vi "TazeASharg.vi"() -> ()   [LabVIEW 2022 SP3]
uses:
  ShargStates.ctl
  ShargTypeDef.ctl
  <vilib>/numeric/Random Number (Range) U64.vi
  <vilib>/numeric/sub_Random U32.vi
  <vilib>/MakerHub/LINX/Public/Utilities/Open Serial.vi
  <vilib>/MakerHub/LINX/Public/Sensors/Motion/Servo/Servo Open One Channel.vi
  <vilib>/MakerHub/LINX/Public/Sensors/Motion/Servo/Servo Close One Channel.vi
  <vilib>/MakerHub/LINX/LMH-LINX.lvlib
  <vilib>/MakerHub/LINX/Public/Sensors/Motion/Servo/Servo.lvlib
panel:
  out "High Scores":string[][](array[string])
  in  "Name":string
  out "Energy":dbl(slide) scale=0.0..100.0
  out "Overheat":bool
  out "Combo":u32
  out "Time":u32
  out "Hit?":bool
  out "Error Out":errorcluster
  out "Cluster Out":T1
  out "Live Score":u32
  out "State":T2=enum."Leaderboard"
  in  "Start Game":bool
  in  "Stop Button":bool
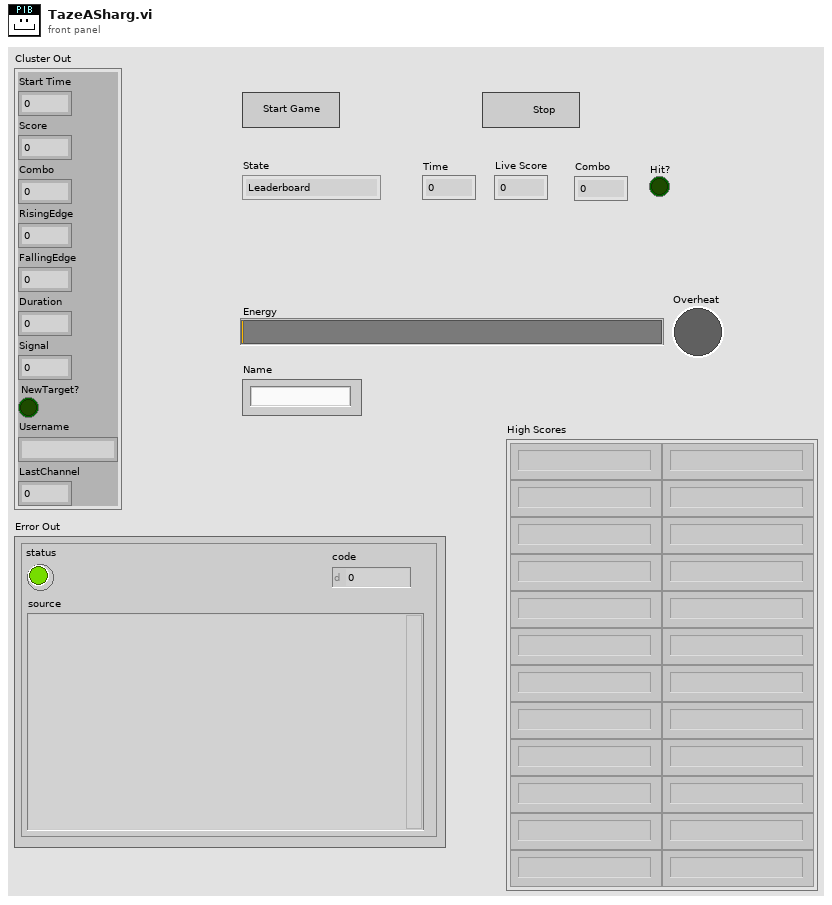
[diagram p1: front panel]
types:
  T1 = typedef "ShargTypeDef.ctl" = cluster{"Start Time":u32, "Score":u32, "Combo":u32, "RisingEdge":u32, "FallingEdge":u32, "Duration":u32, "Signal":i16, "NewTarget?":bool, "Username":string, "LastChannel":i32}
  T2 = typedef "ShargStates.ctl" = enum16{"Initialization", "Leaderboard", "Start Game", "Gameplay", "Update Final Score"}
  T3 = cluster{"Target Up":bool, "Target Start Time":u32, "Target Up Time":u64, "Current Target":u64}
  T4 = cluster{"Laser Pin":u8, "Trigger Pin":u8, "Servo Pin":u8, "Photoresistor Pins":u8[], "RGB LED Pins":u8[]}
  T5 = typedef "LMH-LINX.lvlib/LINX Ref.ctl" = cluster{"IO":T6, "Interface":T7, "LINX Device Config":T8}
  T6 = typedef "LMH-LINX.lvlib/Platform.ctl" = enum16{"Remote", "Local"}
  T7 = typedef "LMH-LINX.lvlib/Interface.ctl" = enum16{"Serial", "TCP"}
  T8 = typedef "LMH-LINX.lvlib/Device.lvlib/LINX Device Config.ctl" = cluster{"Interface":T7, "COM Port":refnum<visa-resource-name>, "TCP Configuration":T9, "Device Family":u8, "Device ID":u8, "Device Name":string, "TCP Ref":refnum<k5>, "Channels":T10}
  T9 = typedef "LMH-LINX.lvlib/Device.lvlib/TCP Config.ctl" = cluster{"IP Address":string, "Port":u16}
  T10 = typedef "LMH-LINX.lvlib/Channels.ctl" = cluster{"DI":u8[], "DO":u8[], "AI":u8[], "AO":u8[], "PWM":u8[], "QE":u8[], "UART":u8[], "I2C 2":u8[], "SPI":u8[], "CAN":u8[], "Servo":u8[], "AI Ref (V)":dbl, "AI Resolution (Bits)":u8, "AO Ref (V)":dbl, "AO Resolution (Bits)":u8}
  T11 = cluster{"Target Up":bool, "millisecond timer value":u32, "number":u64, "Current Target":u64}
  T12 = cluster{"Live Score":u32, "Time":u32, "Combo":u32}
  T13 = enum16{"open", "open or create", "create or replace", "create", "open (read-only)"}
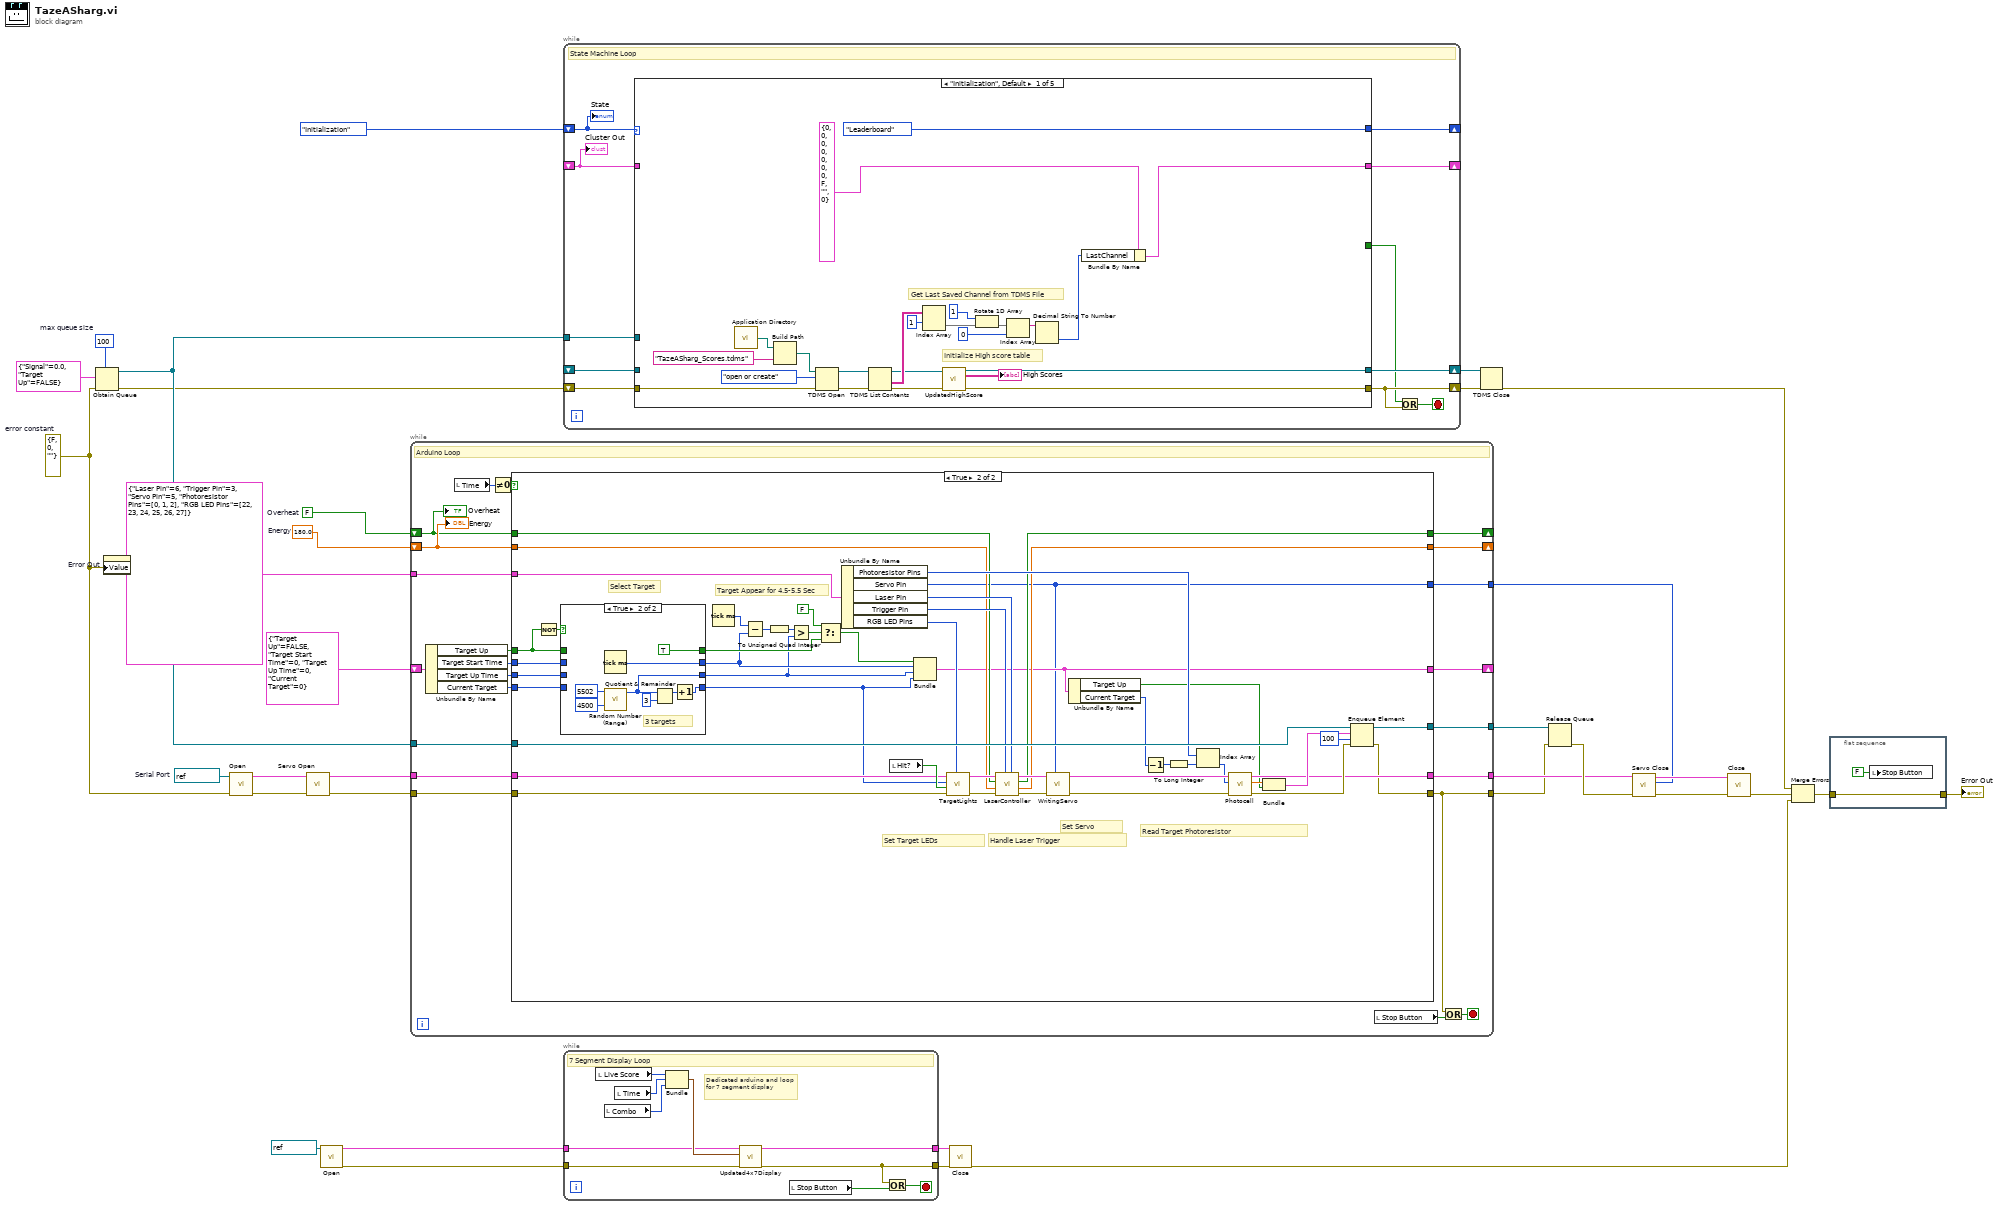
[diagram p0: block diagram]
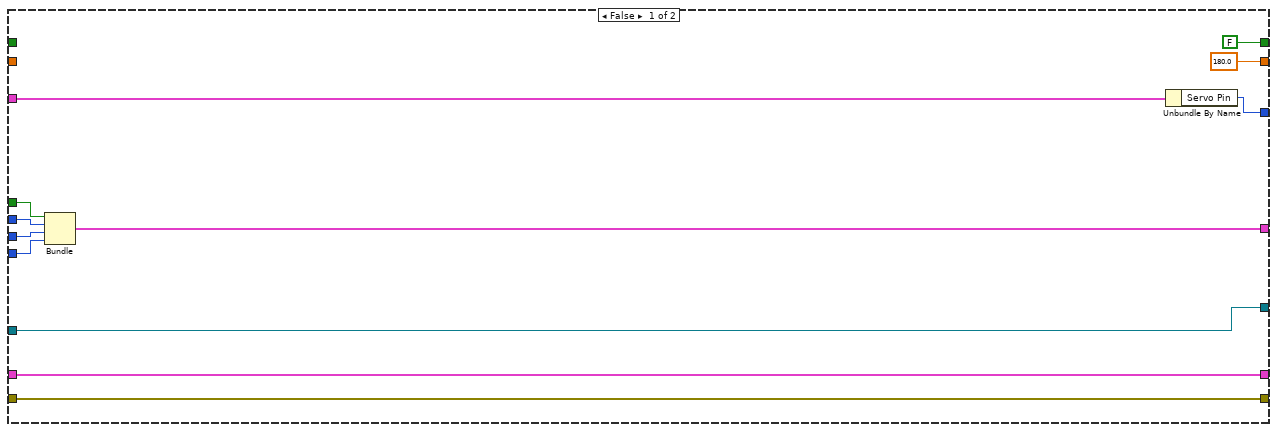
[diagram p2: hidden frame]
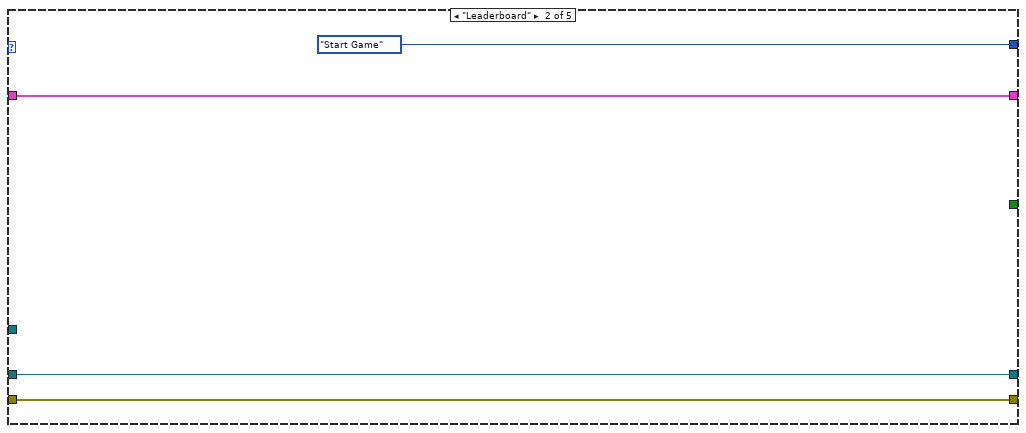
[diagram p4: hidden frame]
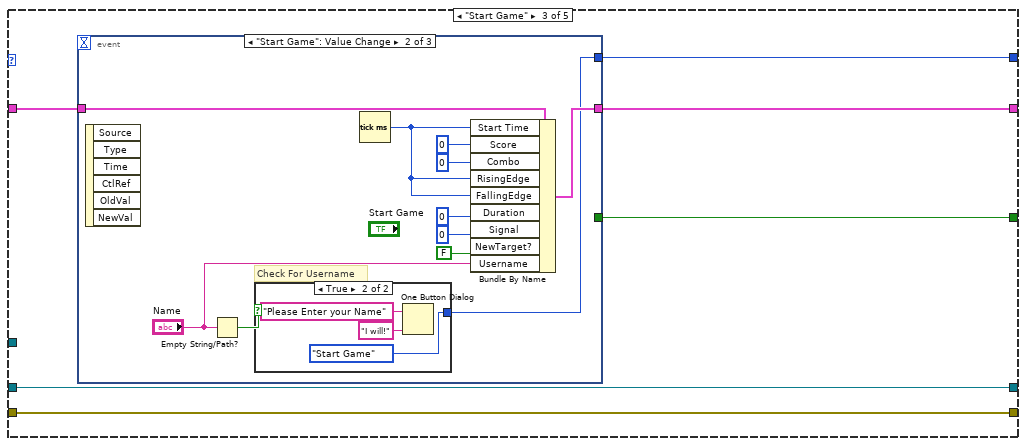
[diagram p5: hidden frame]
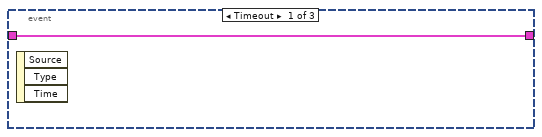
[diagram p6: hidden frame]
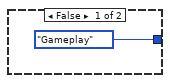
[diagram p7: hidden frame]
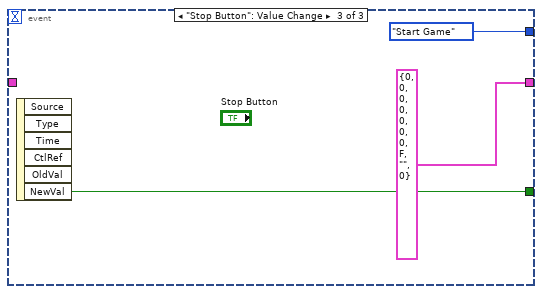
[diagram p8: hidden frame]
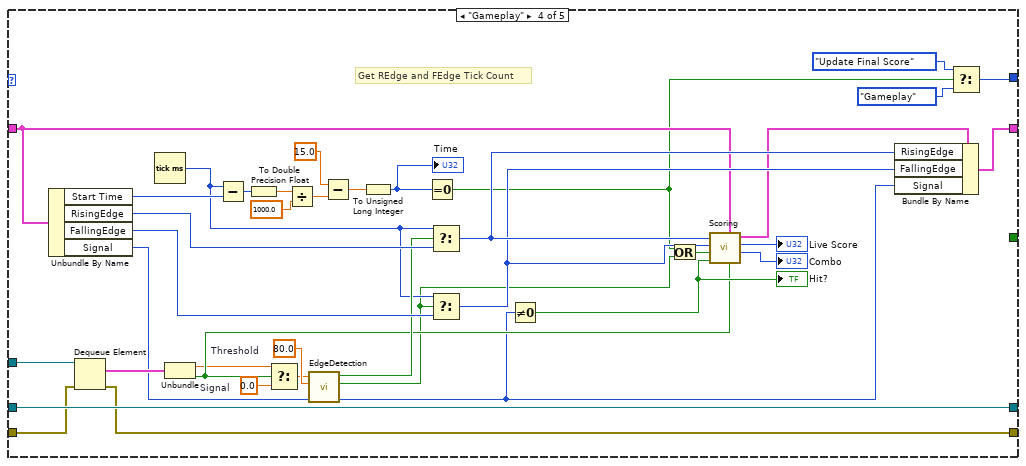
[diagram p9: hidden frame]
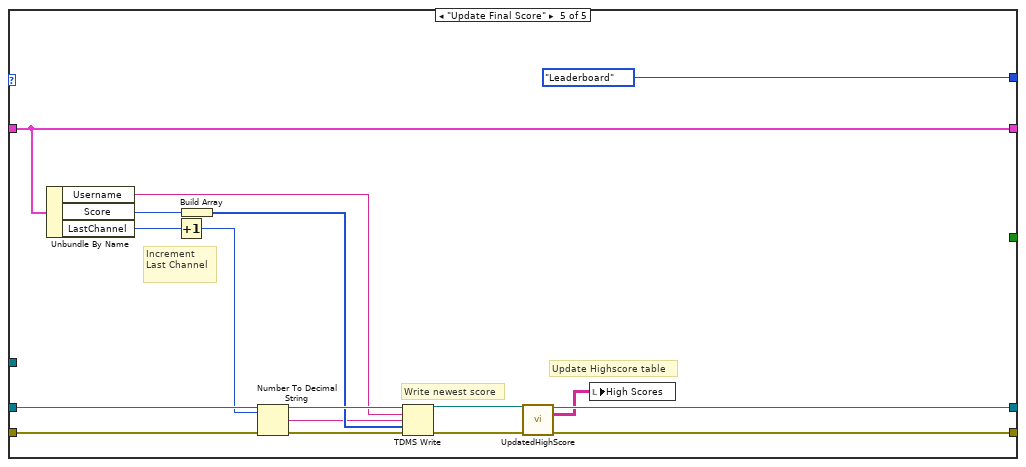
[diagram p10: hidden frame]
diagram:
  w6 = 180.0  # Energy
  w7 = FALSE  # Overheat
  w30 = refnum<visa-resource-name> "COM8"  # Serial Port
  w31 = 100  # max queue size
  w9 = errorcluster {"status"=FALSE, "code"=0, "source"=""}  # error constant
  n1 = Obtain Queue(max queue size (-1, unlimited)=w31, element data type=cluster{"Signal":dbl, "Target Up":bool} {"Signal"=0.0, "Target Up"=FALSE}, error in (no error)=w9) -> (queue out=w33:refnum<queue>, error out=w10:errorcluster)  [unwired: 2 in, 1 out]
  n2 = property on="Error Out" class="Clust (strict)"("Value"=w9) -> ()  [unwired: 2 in, 2 out]
  n3 = call-poly <vilib>:"Open.vi"("Error In"=w9, "Serial Port"=w30) -> ("Error Out"=w27:errorcluster, "LINX Resource"=w29:T5)  [unwired: 7 in, 1 out]
  n4 = call-poly <vilib>:"Servo Open.vi"("Error In"=w27, "LINX Resource"=w29) -> ("Error Out"=w26:errorcluster, "LINX Resource"=w28:T5)  [unwired: 8 in]
  n5 = call-poly <vilib>:"Open.vi"("Serial Port"=refnum<visa-resource-name> "COM5") -> ("Error Out"=w19:errorcluster, "LINX Resource"=w20:T5)  [unwired: 8 in, 1 out]
  n6 = while {
    tunnel: w26 -> [w51]
    tunnel: w28 -> [w52]
    shift-right: [w48] -> _
    shift-left: w7 -> [w45]
    shift-right: [w47] -> _
    shift-left: w6 -> [w46]
    tunnel: w33 -> [w50]
    tunnel: T4 {"Laser Pin"=6, "Trigger Pin"=3, "Servo Pin"=5, "Photoresistor Pins"=[0, 1, 2], "RGB LED Pins"=[22, 23, 24, 25, 26, 27]} -> [w49]
    tunnel: [w44] -> w5
    tunnel: [w35] -> w1
    tunnel: [w43] -> w4
    shift-right: [w37] -> _
    shift-left: T3 {"Target Up"=FALSE, "Target Start Time"=0, "Target Up Time"=0, "Current Target"=0} -> [w42]
    tunnel: [w36] -> w2
    stop <- w54 stop-if-true
    # "Arduino Loop"
    n7 = Unbundle By Name(w42) -> ("Target Up"=w41:bool, "Target Start Time"=w40:u32, "Target Up Time"=w39:u64, "Current Target"=w38:u64)
    n8 = local read "Time"() -> (w56:u32)
    n9 = Not Equal To 0?(x=w56) -> (x != 0?=w55:bool)
    n10 = case shown="True" w55 {
      tunnel: w40 -> [w62 w111]
      tunnel: w41 -> [w63 w110]
      tunnel: w38 -> [w60 w109]
      tunnel: w39 -> [w61 w108]
      tunnel: w52 -> [w65 w92]
      tunnel: w51 -> [w66 w91]
      tunnel: [w65 w90] -> w44
      tunnel: [w66 w89] -> w35
      tunnel: w50 -> [w64 w88]
      tunnel: w49 -> [w58 w86]
      tunnel: w46 -> [_ w81]
      tunnel: w45 -> [_ w80]
      tunnel: [FALSE ("Overheat Out") w79] -> w48
      tunnel: [180.0 ("Energy Out") w78] -> w47
      tunnel: [w64 w77] -> w43
      tunnel: [w59 w72] -> w37
      tunnel: [w57 w70] -> w36
      frame False {
        n11 = Bundle("Target Up"=w63, "Target Start Time"=w62, "Target Up Time"=w61, "Current Target"=w60) -> (w59:T3)  [unwired: 1 in]
        n12 = Unbundle By Name(w58) -> ("Servo Pin"=w57:u8)
      }
      frame True {
        # "Set Servo"
        # "Read Target Photoresistor"
        # "Handle Laser Trigger"
        # "Set Target LEDs"
        # "Target Appear for 4.5-5.5 Sec"
        # "Select Target"
        n13 = Not(x=w110) -> (.not. x?=w107:bool)
        n14 = case shown="True" w107 {
          tunnel: [w119 TRUE] -> w113
          tunnel: [w120 w127] -> w75
          tunnel: [w118 w122] -> w73
          tunnel: w111 -> [w120 _]
          tunnel: w110 -> [w119 _]
          tunnel: w109 -> [w118 _]
          tunnel: [w117 w121] -> w74
          tunnel: w108 -> [w117 _]
          frame False {
          }
          frame True {
            # "3 targets"
            n15 = Tick Count (ms)() -> (millisecond timer value=w127:u32)
            n16 = call-poly <vilib>:"Random Number (Range).vi"("lower bound (0)"=u64 4500, "upper bound (100)"=u64 5502) -> ("number"=w121:u64)  [unwired: 9 in]
            n17 = Quotient & Remainder(x=w121, y=u64 3) -> (x-y*floor(x/y)=w124:u64)  [unwired: 1 out]
            n18 = Increment(x=w124) -> (x+1=w122:u64)
          }
        }
        n19 = Tick Count (ms)() -> (millisecond timer value=w116:u32)
        n20 = Subtract(x=w116, y=w75) -> (x-y=w115:u32)
        n21 = To Unsigned Quad Integer(1:w115) -> (0:w106:u64)
        n22 = Greater?(x=w106, y=w74) -> (0:w114:bool)
        n23 = Select(t=FALSE, s=w114, f=w113) -> (s? t:f=w76:bool)
        n24 = Unbundle By Name(w86) -> ("Photoresistor Pins"=w82:u8[], "Servo Pin"=w70:u8, "Laser Pin"=w83:u8, "Trigger Pin"=w84:u8, "RGB LED Pins"=w85:u8[])
        n25 = local read "Hit?"() -> (w99:bool)
        n26 = Bundle("Target Up"=w76, "millisecond timer value"=w75, "number"=w74, "Current Target"=w73) -> (w72:T11)  [unwired: 1 in]
        n27 = call "TargetLights.vi"("DO Channels"=w85, "Error In"=w91, "Hit?"=w99, "Target Number"=w73, "LINX Resource"=w92) -> ("Error Out"=w96:errorcluster, "LINX Resource 2"=w97:T5)  [unwired: 5 in]
        n28 = call "LaserController.vi"("Laser Pin"=w83, "Trigger Pin"=w84, "Error In"=w96, "Energy In"=w81, "Overheat In"=w80, "LINX Resource In"=w97) -> ("Error Out"=w105:errorcluster, "Energy Out"=w78:dbl, "Overheat Out"=w79:bool, "LINX Resource Out"=w104:T5)  [unwired: 2 in]
        n29 = call "WritingServo.vi"("Servo Pin"=w70, "error in (no error)"=w105, "LINX Resource in"=w104) -> ("error out"=w102:errorcluster, "LINX Resource out"=w101:T5)  [unwired: 7 in]
        n30 = Unbundle By Name(w72) -> ("Target Up"=w69:bool, "Current Target"=w71:u64)
        n31 = Decrement(x=w71) -> (x-1=w100:u64)
        n32 = To Long Integer(number=w100) -> (32bit integer=w98:i32)
        n33 = Index Array(array=w82, index=w98) -> (element=w87:u8)
        n34 = call <vilib>:"Photocell.vi"("Error In"=w102, "AI Channel"=w87, "LINX Resource"=w101) -> ("Error Out"=w103:errorcluster, "Value (0-100)"=w94:dbl, "LINX Resource"=w90:T5)  [unwired: 6 in]
        n35 = Bundle("Value (0-100)"=w94, "Target Up"=w69) -> (w95:cluster{"Value (0-100)":dbl, "Target Up":bool})  [unwired: 1 in]
        n36 = Enqueue Element(queue=w88, element=w95, timeout in ms (-1)=100, error in (no error)=w103) -> (queue out=w77:refnum<queue>, error out=w89:errorcluster)  [unwired: 1 out]
      }
    }
    n37 = local read "Stop Button"() -> (w53:bool)
    n38 = Or(x=w35, y=w53) -> (x .or. y?=w54:bool)
    "Overheat" <- w45
    "Energy" <- w46
  }
  n39 = while {
    tunnel: w20 -> [w134]
    tunnel: w19 -> [w133]
    tunnel: [w132] -> w18
    tunnel: [w130] -> w17
    stop <- w131 stop-if-true
    # "Dedicated arduino and loop for 7 segment display"
    # "7 Segment Display Loop"
    n40 = local read "Live Score"() -> (w138:u32)
    n41 = local read "Combo"() -> (w136:u32)
    n42 = local read "Time"() -> (w137:u32)
    n43 = Bundle("Live Score"=w138, "Time"=w137, "Combo"=w136) -> (w135:T12)  [unwired: 1 in]
    n44 = call "Updated4x7Display.vi"("Error In"=w133, "Cluster"=w135, "LINX Resource In"=w134) -> ("Error Out"=w130:errorcluster, "LINX Resource Out"=w132:T5)  [unwired: 7 in]
    n45 = local read "Stop Button"() -> (w129:bool)
    n46 = Or(x=w130, y=w129) -> (x .or. y?=w131:bool)
  }
  n47 = while {
    shift-right: [w148] -> _
    shift-left: ShargStates."Initialization" -> [w149]
    shift-right: [w147] -> _
    shift-left: _ -> [w146]
    tunnel: w33 -> [w145]
    shift-right: [w143] -> w16
    shift-left: _ -> [w142]
    shift-right: [w140] -> w15
    shift-left: w10 -> [w141]
    stop <- w144 stop-if-true
    # "State Machine Loop"
    n48 = case shown="\"Initialization\", Default" w149 {
      tunnel: [ShargStates."Leaderboard" ShargStates."Start Game" w182 w239 ShargStates."Leaderboard"] -> w148
      tunnel: [w150 w175 w180 w202 w253] -> w147
      tunnel: w146 -> [_ w175 w181 w227 w253]
      tunnel: w145 -> [_ _ _ w236 _]
      tunnel: [w153 w173 w179 w203 w242] -> w140
      tunnel: [w155 w174 w177 w208 w243] -> w143
      tunnel: w142 -> [_ w174 w177 w208 w252]
      tunnel: w141 -> [w168 w173 w179 w204 w251]
      tunnel: [_ _ w178 _ _] -> w139
      frame "Initialization", Default {
        # "Get Last Saved Channel from TDMS File"
        # "Initialize High score table"
        n49 = call <vilib>:"Application Directory.vi"() -> ("Application Directory"=w171:path)
        n50 = Build Path(base path=w171, name or relative path="TazeASharg_Scores.tdms") -> (appended path=w170:path)
        n51 = TDMS Open(8:w168, 10:T13."open or create" ("operation (0:open)"), 11:w170) -> (0:w166:errorcluster, 3:w167:refnum<k34>)  [unwired: 4 in]
        n52 = TDMS List Contents(4:w166, 7:w167) -> (0:w152:errorcluster, 1:w160:string[][], 3:w156:refnum<k34>)  [unwired: 1 in, 1 out]
        n53 = Index Array(array=w160, index (row)=1) -> (element=w165:string[])  [unwired: 1 in]
        n54 = call "UpdatedHighScore.vi"("tdms file"=w156, "error in (no error)"=w152) -> ("tdms file out"=w155:refnum<k34>, "Array"=→"High Scores":string[][], "error out"=w153:errorcluster)  [unwired: 11 in]
        n55 = Rotate 1D Array(1:w165, 2:1 ("n")) -> (0:w163:string[])
        n56 = Index Array(array=w163, index=0) -> (element=w159:string)
        n57 = Decimal String To Number(string=w159) -> (number=w157:i32)  [unwired: 2 in, 1 out]
        n58 = Bundle By Name(cluster=T1 {"Start Time"=0, "Score"=0, "Combo"=0, "RisingEdge"=0, "FallingEdge"=0, "Duration"=0, "Signal"=0, "NewTarget?"=FALSE, "Username"="", "LastChannel"=0} ("Cluster"), "LastChannel"=w157) -> (w150:T1)
      }
      frame "Leaderboard" {
      }
      frame "Start Game" {
        n59 = event shown="[1] \"Start Game\": Value Change" {
          selector: _ -> [_ _ _]
          dyn-events: _ -> [_ _ _]
          timeout: _ -> [_ _ _]
          tunnel: [_ w185 ShargStates."Start Game"] -> w182
          tunnel: w181 -> [w183 w194 _]
          tunnel: [w183 w193 T1 {"Start Time"=0, "Score"=0, "Combo"=0, "RisingEdge"=0, "FallingEdge"=0, "Duration"=0, "Signal"=0, "NewTarget?"=FALSE, "Username"="", "LastChannel"=0} ("Cluster Out")] -> w180
          tunnel: [_ _ w199] -> w178
          event Timeout {
            n60 = event-data() -> ()  [unwired: 1 in, 3 out]
          }
          event "Start Game": Value Change {
            # "Check For Username"
            n61 = event-data() -> ()  [unwired: 1 in, 6 out]
            n62 = Empty String/Path?(string/path="Name") -> (empty?=w186:bool)
            n63 = case shown="True" w186 {
              tunnel: [ShargStates."Gameplay" ShargStates."Start Game"] -> w185
              frame False {
              }
              frame True {
                n64 = One Button Dialog(message="Please Enter your Name", button name ("OK")="I will!") -> ()  [unwired: 1 out]
              }
            }
            n65 = Tick Count (ms)() -> (millisecond timer value=w187:u32)
            n66 = Bundle By Name(cluster=w194, "Start Time"=w187, "Score"=u32 0, "Combo"=u32 0, "RisingEdge"=w187, "FallingEdge"=w187, "Duration"=u32 0, "Signal"=i16 0, "NewTarget?"=FALSE, "Username"="Name") -> (w193:T1)
          }
          event "Stop Button": Value Change {
            n67 = event-data() -> ("NewVal"=w199:bool)  [unwired: 1 in, 5 out]
          }
        }
      }
      frame "Gameplay" {
        w229 = 0.0  # Signal
        w235 = 80.0  # Threshold
        # "Get REdge and FEdge Tick Count"
        n68 = Unbundle By Name(w227) -> ("Start Time"=w225:u32, "RisingEdge"=w232:u32, "FallingEdge"=w231:u32, "Signal"=w211:i16)
        n69 = Dequeue Element(queue=w236, error in (no error)=w204) -> (element=w226:cluster{"Signal":dbl, "Target Up":bool}, error out=w203:errorcluster)  [unwired: 1 in, 2 out]
        n70 = Tick Count (ms)() -> (millisecond timer value=w224:u32)
        n71 = Unbundle(w226) -> ("Signal"=w213:dbl, "Target Up"=w214:bool)
        n72 = Subtract(x=w224, y=w225) -> (x-y=w223:u32)
        n73 = To Double Precision Float(number=w223) -> (double precision float=w221:dbl)
        n74 = Select(t=w213, s=w214, f=w229) -> (s? t:f=w212:dbl)
        n75 = Divide(x=w221, y=1000.0) -> (x/y=w220:dbl)
        n76 = call "EdgeDetection.vi"("Previous Value"=w211, "Threshold"=w235, "Analog Input"=w212) -> ("Digitized"=w210:i16, "Falling Edge"=w206:bool, "Rising Edge"=w230:bool)  [unwired: 4 in]
        n77 = Subtract(x=15.0, y=w220) -> (x-y=w216:dbl)
        n78 = To Unsigned Long Integer(number=w216) -> (unsigned 32bit integer=w209:u32)
        "Time" <- w209
        n79 = Equal To 0?(x=w209) -> (x = 0?=w207:bool)
        n80 = Select(t=w224, s=w230, f=w232) -> (s? t:f=w234:u32)
        n81 = Select(t=w224, s=w206, f=w231) -> (s? t:f=w233:u32)
        n82 = Not Equal To 0?(x=w210) -> (x != 0?=w215:bool)
        "Hit?" <- w215
        n83 = Or(x=w207, y=w206) -> (x .or. y?=w205:bool)
        n84 = call "Scoring.vi"("RisingEdge"=w234, "FallingEdge"=w233, "FallingEdge?"=w205, "Hit?"=w215, "Cluster In"=w227, "TargetUp?"=w214) -> ("Cluster Out"=w228:T1, "Live Score"=→"Live Score":u32, "Combo"=→"Combo":u32)  [unwired: 2 in]
        n85 = Bundle By Name(cluster=w228, "RisingEdge"=w234, "FallingEdge"=w233, "Signal"=w210) -> (w202:T1)
        n86 = Select(t=ShargStates."Update Final Score", s=w207, f=ShargStates."Gameplay") -> (s? t:f=w239:T2)
      }
      frame "Update Final Score" {
        # "Write newest score"
        # "Update Highscore table"
        # "Increment Last Channel"
        n87 = Unbundle By Name(w253) -> ("Username"=w246:string, "Score"=w250:u32, "LastChannel"=w245:i32)
        n88 = Increment(x=w245) -> (x+1=w247:i32)
        n89 = Build Array(w250) -> (w249:u32[])
        n90 = Number To Decimal String(number=w247) -> (decimal integer string=w248:string)  [unwired: 1 in]
        n91 = TDMS Write(0:w252, 5:w246, 7:w248, 9:w249, 11:w251) -> (4:w244:refnum<k34>, 15:w241:errorcluster)  [unwired: 1 in, 2 out]
        n92 = call "UpdatedHighScore.vi"("tdms file"=w244, "error in (no error)"=w241) -> ("tdms file out"=w243:refnum<k34>, "Array"=w240:string[][], "error out"=w242:errorcluster)  [unwired: 11 in]
        n93 = local write "High Scores"(w240) -> ()
      }
    }
    n94 = Or(x=w139, y=w140) -> (x .or. y?=w144:bool)
    "State" <- w149
    "Cluster Out" <- w146
  }
  n95 = call <vilib>:"Close.vi"("Error In"=w17, "LINX Resource"=w18) -> ("Error Out"=w11:errorcluster)  [unwired: 9 in]
  n96 = TDMS Close(8:w15, 11:w16) -> (0:w12:errorcluster)  [unwired: 1 out]
  n97 = Release Queue(queue=w4, error in (no error)=w1) -> (error out=w23:errorcluster)  [unwired: 1 in, 2 out]
  n98 = call-poly <vilib>:"Servo Close.vi"("Error In"=w23, "Servo Channel"=w2, "LINX Resource"=w5) -> ("Error Out"=w24:errorcluster, "LINX Resource"=w25:T5)  [unwired: 7 in]
  n99 = call <vilib>:"Close.vi"("Error In"=w24, "LINX Resource"=w25) -> ("Error Out"=w14:errorcluster)  [unwired: 9 in]
  n100 = Merge Errors(w12, w14, w11) -> (w13:errorcluster)
  n101 = flat-sequence {
    tunnel: w13 -> [w255]
    tunnel: [w255] -> w22
    frame #0 {
      n102 = local write "Stop Button"(FALSE ("Stop Button")) -> ()
    }
  }
  "Error Out" <- w22
